vi "CleanUp.vi"(0 "object in":refnum<class "Modbus.lvclass">, 5 "error in (no error)":errorcluster) -> (14 "object out":refnum<class "Modbus.lvclass">, 19 "error out":errorcluster)   [LabVIEW 2023, in "HardwareAbstractionLayer_LVOOP.lvlib" / "Modbus.lvclass"]
uses:
  Modbus.lvclass
  Modbus.lvclass/Modbus.ctl
  <vilib>/NI/Modbus Library/API/Master/Modbus Master.lvclass
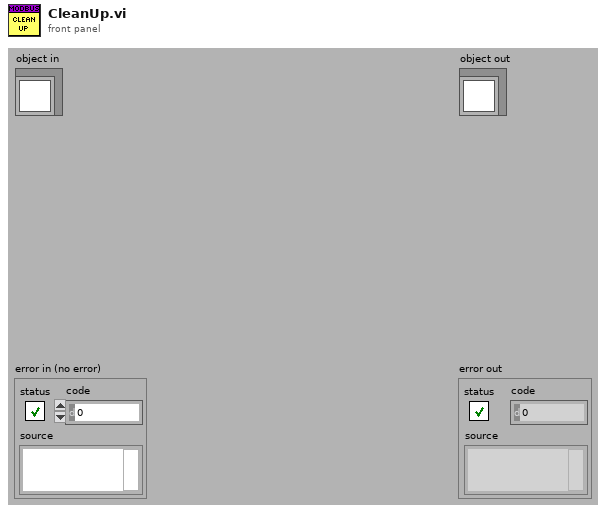
[diagram p1: front panel]
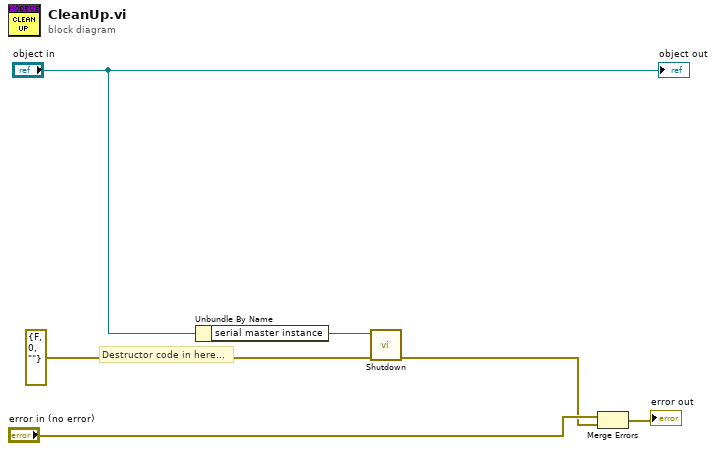
[diagram p0: block diagram]
diagram:
  # "Destructor code in here..."
  n1 = Unbundle By Name("object in") -> ("serial master instance"=w3:refnum<class "Modbus Master.lvclass">)
  n2 = call-dynamic "Shutdown.vi"("error in"=errorcluster {"status"=FALSE, "code"=0, "source"=""} ("error in (no error)"), "Modbus master in"=w3) -> ("error out"=w1:errorcluster)  [unwired: 9 in]
  n3 = Merge Errors("error in (no error)", w1) -> (→"error out":errorcluster)
  "object out" <- "object in"
